vi "数据库写入.vi"(0 "pH":dbl format="%.2f", 1 "DO":dbl format="%.2f", 2 "ORP":dbl format="%.2f", 3 "NH4N":dbl format="%.2f", 4 "CODMn":dbl format="%.2f", 5 "error in (no error)":errorcluster caption="错误输入（无错误）") -> (14 "表格":string[][](table), 19 "error out":errorcluster caption="错误输出")   [LabVIEW 2016, in "数据传输系统-02.lvlib"]
uses:
  <vilib>/Utility/sysdir.llb/System Directory Type.ctl
  <vilib>/addons/database/Connection.llb/DB Tools Open Connec (String).vi
  <vilib>/addons/database/_DB Variant To Data/Database Variant To Data.xnode
  <vilib>/addons/database/NI_Database_API.lvlib
panel:
  in  "Delay Time (s)":dbl=10.0 caption="延迟时间(s)"
  in  "poll":bool
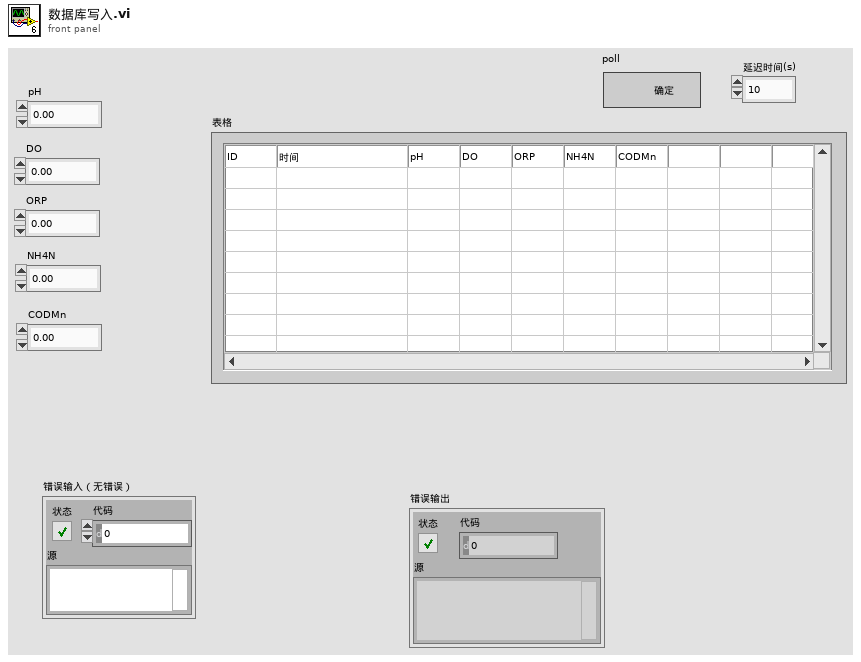
[diagram p1: front panel]
types:
  T1 = typedef "System Directory Type.ctl" = i32
  T2 = typedef "NI_Database_API.lvlib/Conn ObjectReference.ctl" = refnum<k1>
  T3 = cluster{"date/time string":string, string, string, string, string, string}
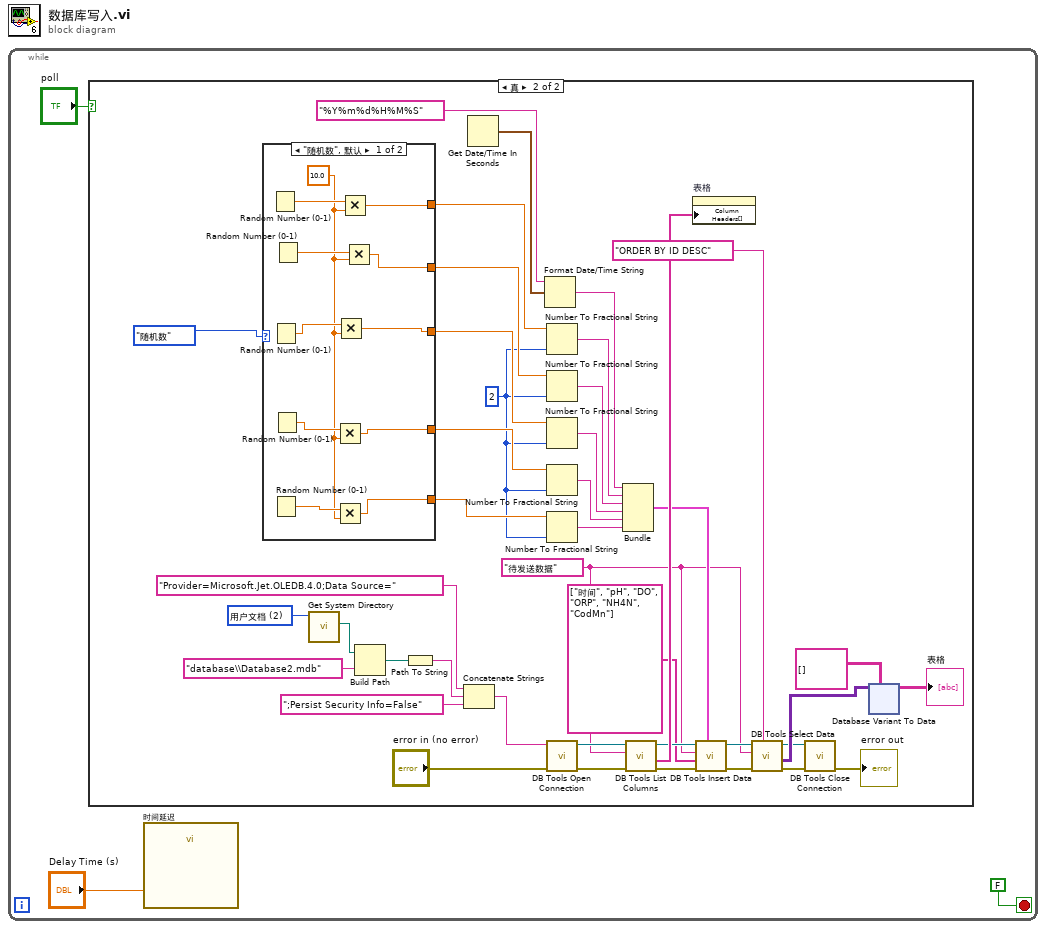
[diagram p0: block diagram]
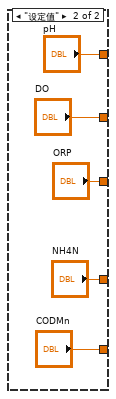
[diagram p3: hidden frame]
diagram:
  n1 = while {
    stop <- FALSE stop-if-true
    n2 = case shown="真" "poll" {
      frame False {
      }
      frame True {
        w12 = T1 2 items=["用户目录"=0, "用户桌面"=1, "用户文档"=2, "用户应用程序数据"=3, "用户设置"=4, "用户临时目录"=5, "公共文档"=6, "公共应用程序数据"=7, "公共设置"=8, "公共缓存"=13, "系统核心库"=9, "系统安装库"=10, "应用程序文件"=11, "启动盘根目录"=12] ("system directory type")
        w13 = "待发送数据" ("组合框")
        w21 = i16 2 ("精度(6)")
        n3 = case shown="\"随机数\", 默认" enum16{"随机数", "设定值"}."随机数" {
          tunnel: [w54 "pH"] -> w26
          tunnel: [w48 "DO"] -> w25
          tunnel: [w47 "ORP"] -> w24
          tunnel: [w46 "NH4N"] -> w23
          tunnel: [w45 "CODMn"] -> w22
          frame "随机数", Default {
            w49 = 10.0 ("y")
            n4 = Random Number (0-1)() -> (number: 0 to 1=w55:dbl)
            n5 = Random Number (0-1)() -> (number: 0 to 1=w51:dbl)
            n6 = Random Number (0-1)() -> (number: 0 to 1=w53:dbl)
            n7 = Random Number (0-1)() -> (number: 0 to 1=w52:dbl)
            n8 = Random Number (0-1)() -> (number: 0 to 1=w50:dbl)
            n9 = Multiply(x=w52, y=w49) -> (x*y=w46:dbl)
            n10 = Multiply(x=w53, y=w49) -> (x*y=w45:dbl)
            n11 = Multiply(x=w51, y=w49) -> (x*y=w47:dbl)
            n12 = Multiply(x=w55, y=w49) -> (x*y=w54:dbl)
            n13 = Multiply(x=w50, y=w49) -> (x*y=w48:dbl)
          }
          frame "设定值" {
          }
        }
        n14 = call <vilib>:"Get System Directory.vi"("system directory type"=w12) -> ("system directory"=w10:path)  [unwired: 10 in]
        n15 = Build Path(base path=w10, name or relative path="database\\Database2.mdb" ("condition")) -> (appended path=w9:path)
        n16 = Path To String(path=w9) -> (string=w8:string)
        n17 = Concatenate Strings("Provider=Microsoft.Jet.OLEDB.4.0;Data Source=" ("condition"), w8, ";Persist Security Info=False" ("condition")) -> (w6:string)
        n18 = Get Date/Time In Seconds() -> (seconds since 1Jan1904=w28:timestamp)
        n19 = Format Date/Time String(time format string (%c)="%Y%m%d%H%M%S" ("时间格式字符串(%c)"), seconds (now)=w28) -> (date/time string=w19:string)  [unwired: 1 in]
        n20 = Number To Fractional String(number=w26, precision (6)=w21) -> (F-format string=w18:string)  [unwired: 2 in]
        n21 = Number To Fractional String(number=w25, precision (6)=w21) -> (F-format string=w17:string)  [unwired: 2 in]
        n22 = Number To Fractional String(number=w24, precision (6)=w21) -> (F-format string=w16:string)  [unwired: 2 in]
        n23 = Number To Fractional String(number=w23, precision (6)=w21) -> (F-format string=w15:string)  [unwired: 2 in]
        n24 = Number To Fractional String(number=w22, precision (6)=w21) -> (F-format string=w14:string)  [unwired: 2 in]
        n25 = call-poly <vilib>:"DB Tools Open Connection.vi"("error in (no error)"="error in (no error)", "connection information"=w6) -> ("error out"=w37:errorcluster, "connection reference"=w36:T2)  [unwired: 6 in]
        n26 = Bundle("date/time string"=w19, w18, w17, w16, w15, w14) -> (w20:T3)  [unwired: 1 in]
        n27 = call <vilib>:"DB Tools List Columns.vi"("error in (no error)"=w37, "table"=w13, "connection reference"=w36) -> ("error out"=w33:errorcluster, "columns"=w38:string[], "connection reference out"=w32:T2)  [unwired: 1 in, 1 out]
        n28 = property on="表格" class="Tbl (严格)"("Column Headers[]"=w38) -> ()  [unwired: 2 in, 2 out]
        n29 = call <vilib>:"DB Tools Insert Data.vi"("data"=w20, "error in (no error)"=w33, "columns"=string[] ["时间", "pH", "DO", "ORP", "NH4N", "CodMn"], "table"=w13, "connection reference"=w32) -> ("error out"=w30:errorcluster, "connection reference out"=w31:T2)  [unwired: 5 in]
        n30 = call <vilib>:"DB Tools Select Data.vi"("condition"="ORDER BY ID DESC", "error in (no error)"=w30, "table"=w13, "connection reference"=w31) -> ("error out"=w34:errorcluster, "data"=w44:variant[][], "connection reference out"=w35:T2)  [unwired: 2 in]
        n31 = call <vilib>:"DB Tools Close Connection.vi"("error in (no error)"=w34, "connection reference"=w35) -> ("error out"=→"error out":errorcluster)  [unwired: 5 in]
        n32 = xnode "Database Variant To Data"("database variant"=w44, "type"=string[][] []) -> ("data"=→"表格":string[][])  [unwired: 1 in, 1 out]
      }
    }
    n33 = call "时间延迟"("Delay Time (s)"="Delay Time (s)") -> ()  [unwired: 10 in, 1 out]
  }
